vi "CRISTALIZADOR_COMM.vi"(8 "error in (no error)":errorcluster) -> (0 "error out":errorcluster, 2 "Cancelled?":bool, 3 "Comunicaciones":T1={"IKA_Eurostar"="", "IKA"=FALSE, "Agilent"="ASRL6::INSTR", "AGL"=FALSE, "SLOT AGL"=TRUE})   [LabVIEW 2017]
doc: "Use this template to create a dialog box. This template polls the state of the buttons on the front panel and does not use events. Use the Dialog Using Events template (not available in Base package) to create a dialog box with event handling."
uses:
  CRISTALIZADOR_COMM.ctl
panel:
  in  "SLOT AGL":bool caption="Checkbox"
  in  "AGL":bool=TRUE caption="Checkbox"
  in  "Agilent":refnum<visa-resource-name>="COM1"
  in  "IKA":bool=TRUE caption="Checkbox"
  in  "IKA_Eurostar":refnum<visa-resource-name>="COM3"
  out "Si usado":bool=TRUE caption="Checkbox"
  out "No usado":bool=TRUE caption="Checkbox"
  in  "Cancel Button":bool
  in  "OK Button":bool
  # "Puertos serie ..."
  # "asslcdms Feb2023 LV17"
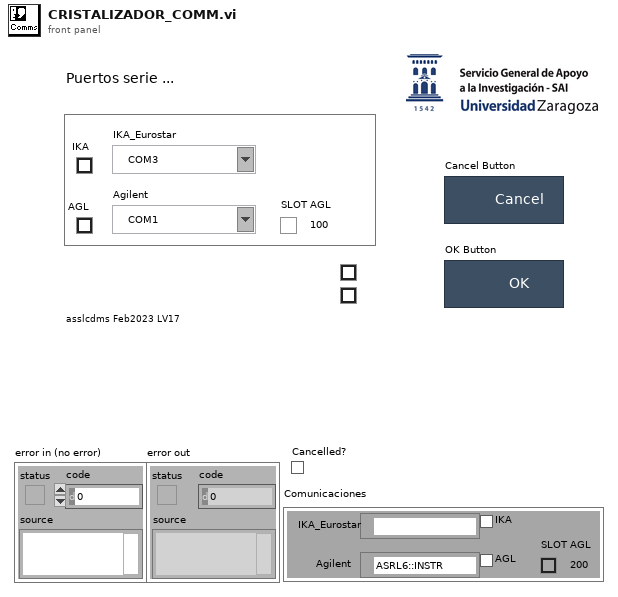
[diagram p1: front panel]
types:
  T1 = typedef "CRISTALIZADOR_COMM.ctl" = cluster{"IKA_Eurostar":refnum<visa-resource-name>, "IKA":bool, "Agilent":refnum<visa-resource-name>, "AGL":bool, "SLOT AGL":bool}
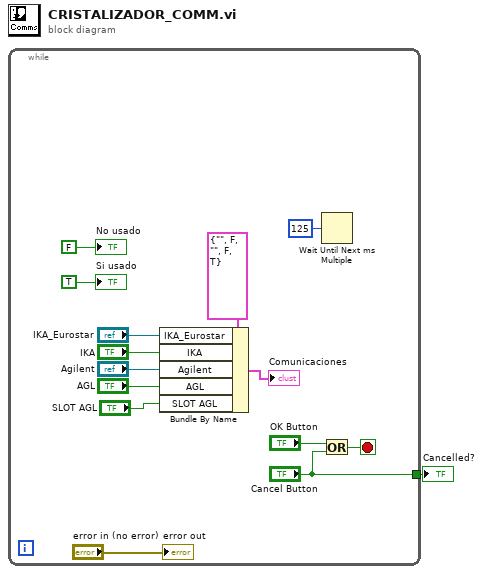
[diagram p0: block diagram]
diagram:
  n1 = while {
    tunnel: ["Cancel Button"] -> w1
    stop <- w14 stop-if-true
    n2 = Bundle By Name(cluster=T1 {"IKA_Eurostar"="", "IKA"=FALSE, "Agilent"="", "AGL"=FALSE, "SLOT AGL"=TRUE} ("Comunicaciones"), "IKA_Eurostar"="IKA_Eurostar", "IKA"="IKA", "Agilent"="Agilent", "AGL"="AGL", "SLOT AGL"="SLOT AGL") -> (→"Comunicaciones":T1)
    n3 = Wait Until Next ms Multiple(millisecond multiple=u32 125) -> ()  [unwired: 1 out]
    n4 = Or(x="OK Button", y="Cancel Button") -> (x .or. y?=w14:bool)
    "error out" <- "error in (no error)"
    "No usado" <- FALSE ("No usado")
    "Si usado" <- TRUE ("Si usado")
  }
  "Cancelled?" <- w1
